vi "计算两条直线距离.vi"(8 "Img in":T1, 10 "Straight Edge (下直线)":T2, 11 "Straight Edge (上直线)":T2) -> (3 "Distance":dbl)   [LabVIEW 2014]
uses:
  <vilib>/vision/Image Controls.llb/IMAQ Image.ctl
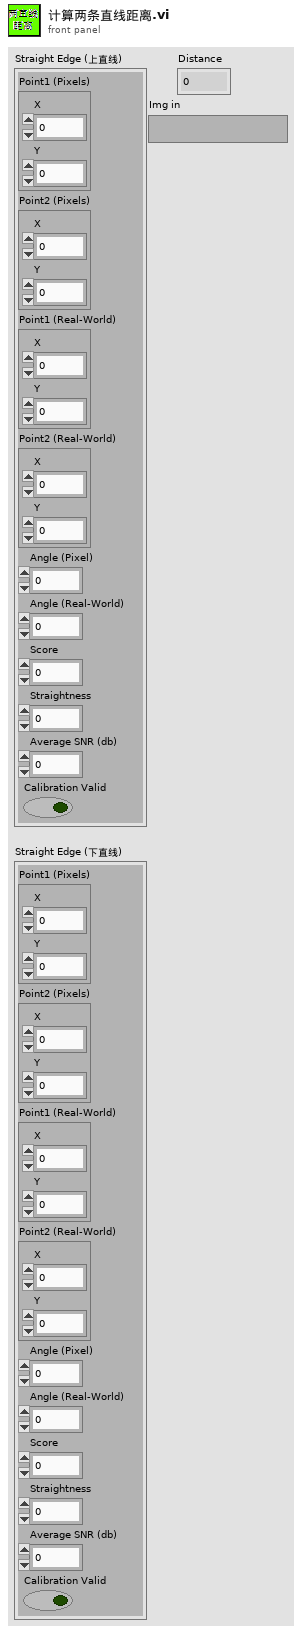
[diagram p1: front panel]
types:
  T1 = typedef "IMAQ Image.ctl" = refnum<image>
  T2 = cluster{"Point1 (Pixels)":cluster{"X":sgl, "Y":sgl}, "Point2 (Pixels)":cluster{"X":sgl, "Y":sgl}, "Point1 (Real-World)":cluster{"X":sgl, "Y":sgl}, "Point2 (Real-World)":cluster{"X":sgl, "Y":sgl}, "Angle (Pixel)":dbl, "Angle (Real-World)":dbl, "Score":dbl, "Straightness":dbl, "Average SNR (db)":dbl, "Calibration Valid":bool}
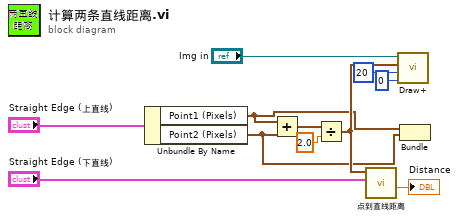
[diagram p0: block diagram]
diagram:
  n1 = Unbundle By Name("Straight Edge (上直线)") -> ("Point1 (Pixels)"=w4:cluster{"X":sgl, "Y":sgl}, "Point2 (Pixels)"=w3:cluster{"X":sgl, "Y":sgl})
  n2 = Add(x=w4, y=w3) -> (x+y=w8:cluster{"X":sgl, "Y":sgl})
  n3 = Divide(x=w8, y=2.0) -> (x/y=w6:cluster{"X":dbl, "Y":dbl})
  n4 = call "点到直线距离.vi"("Straight Edge (X)"="Straight Edge (下直线)", "簇"=w6) -> ("Distance"=→"Distance":dbl)  [unwired: 7 in, 2 out]
  n5 = call "Draw+.vi"("Pos_Y"=0 ("H"), "Pos_X"=20 ("W"), "input cluster"=w6, "Image In"="Img in") -> ()  [unwired: 2 in, 1 out]
  n6 = Bundle("Point1 (Pixels)"=w4, "Point2 (Pixels)"=w3) -> ()  [unwired: 1 in, 1 out]
